vi "ACR_Connect_configTerminal.vi"() -> ()   [LabVIEW 2015]
uses:
  <vilib>/Instr/_visa.llb/VISA Configure Serial Port (Instr).vi
panel:
  in  "nPort":i32=28
  out "Speed Out":dbl
  out "Torque Out":dbl
  out "Running LED":bool
  in  "baud rate":u16(ring)=19200 items=["300"=300, "600"=600, "1200"=1200, "2400"=2400, "4800"=4800, "9600"=9600, "19200"=19200, "38400"=38400]
  in  "flow control":u16(ring) items=["None"=0, "XON/XOFF"=1, "RTS/CTS"=2, "DTR/DSR"=4]
  in  "stop bits":u16(ring)=10 items=["1.0"=10, "1.5"=15, "2.0"=20]
  in  "parity":u16(ring) items=["None", "Odd", "Even", "Mark", "Space"]
  in  "data bits":u16=8 min=5 max=8 step=1
  in  "VISA Refnum in":refnum<visa-resource-name>="COM5"
  in  "Reset Graph":bool
  in  "Sampling Time (s)":dbl=0.2
  out "Read result 2":dbl
  in  "Target":string="p12289"
  out "XY Graph":cluster{dbl[], dbl[]}[](graph)
  out "Read result":dbl
  out "Read error out":errorcluster
  in  "Read error in \n(no error)":errorcluster
  in  "Actual":string="p38144"
  in  "Move CMD":string="x/100"
  in  "OK Button":bool
  in  "Write String Array":string[](array[string])=["detach all", "new all", "clear", "attach master0", "attach slave0 axis0 \"x\"", "axis0 drive on"]
  out "Terminal Status":bool
  in  "ComACRServerLib.IChannel":refnum<k7>
  in  "bstrIP Property":string="192.168.10.40"
  out "Connect error out":errorcluster
  in  "Connect error in \n(no error)":errorcluster
  # "Ethernet Configuration"
  # "Command"
  # "Configure"
  # "detach all\nnew all\nclear\nattach master0\nattach slave0 axis0 \"x\"\naxis0 drive on"
  # "Read P Parameter"
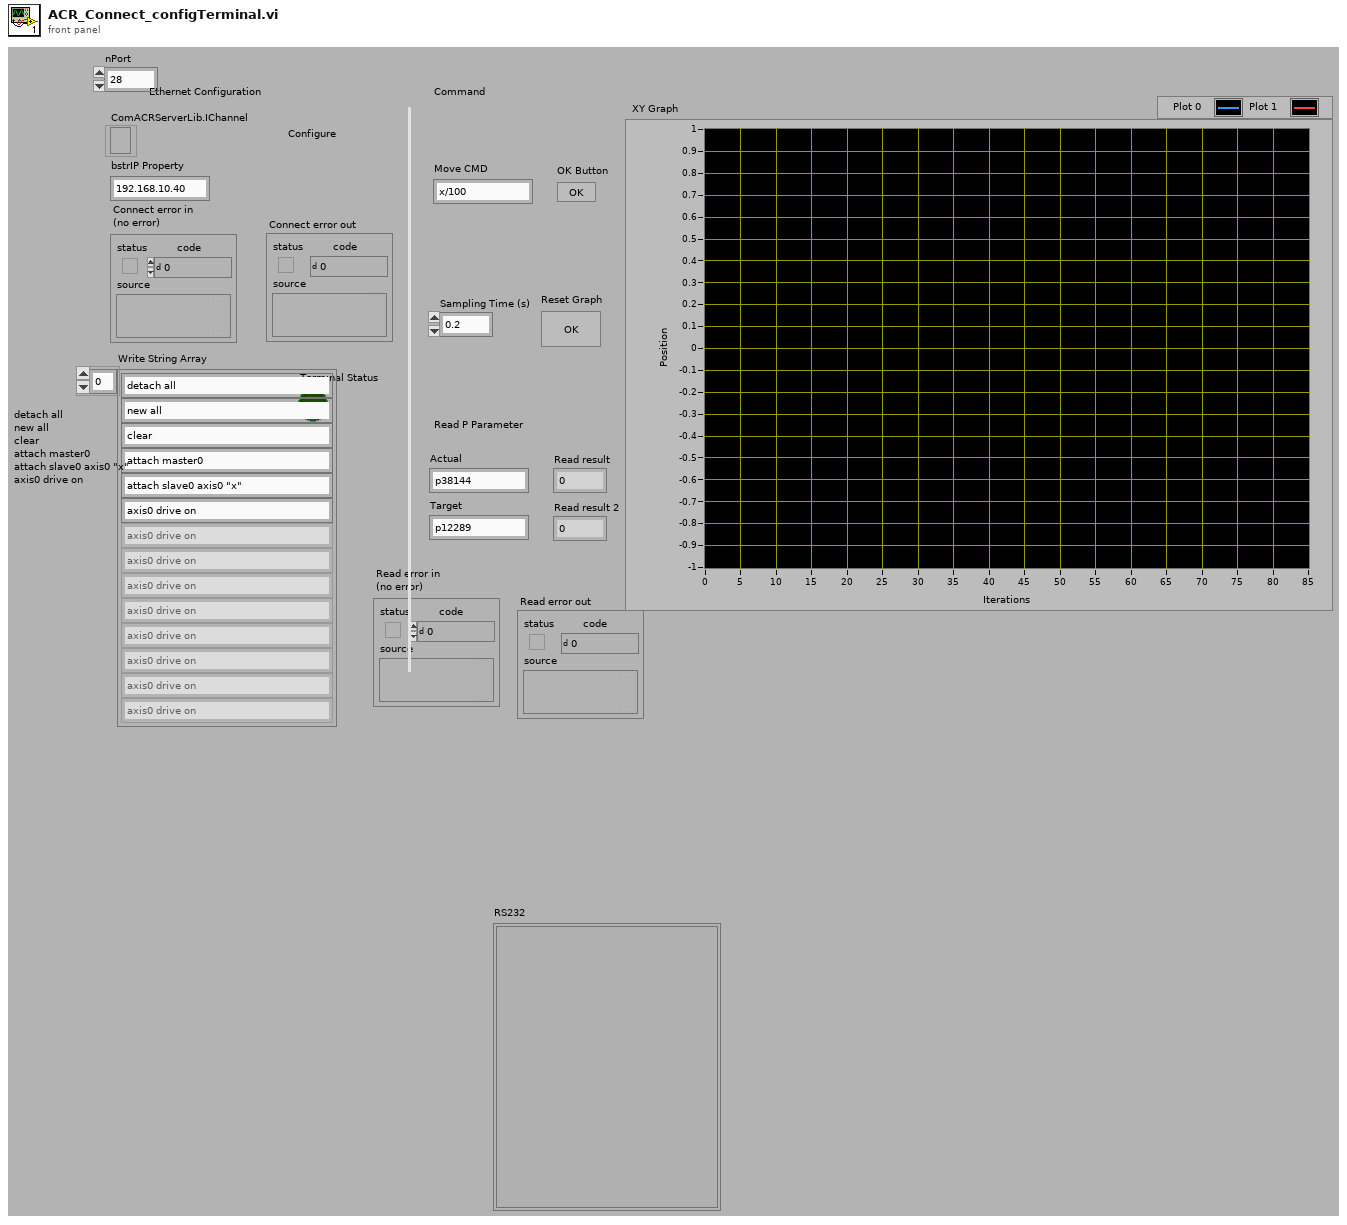
[diagram p1: front panel]
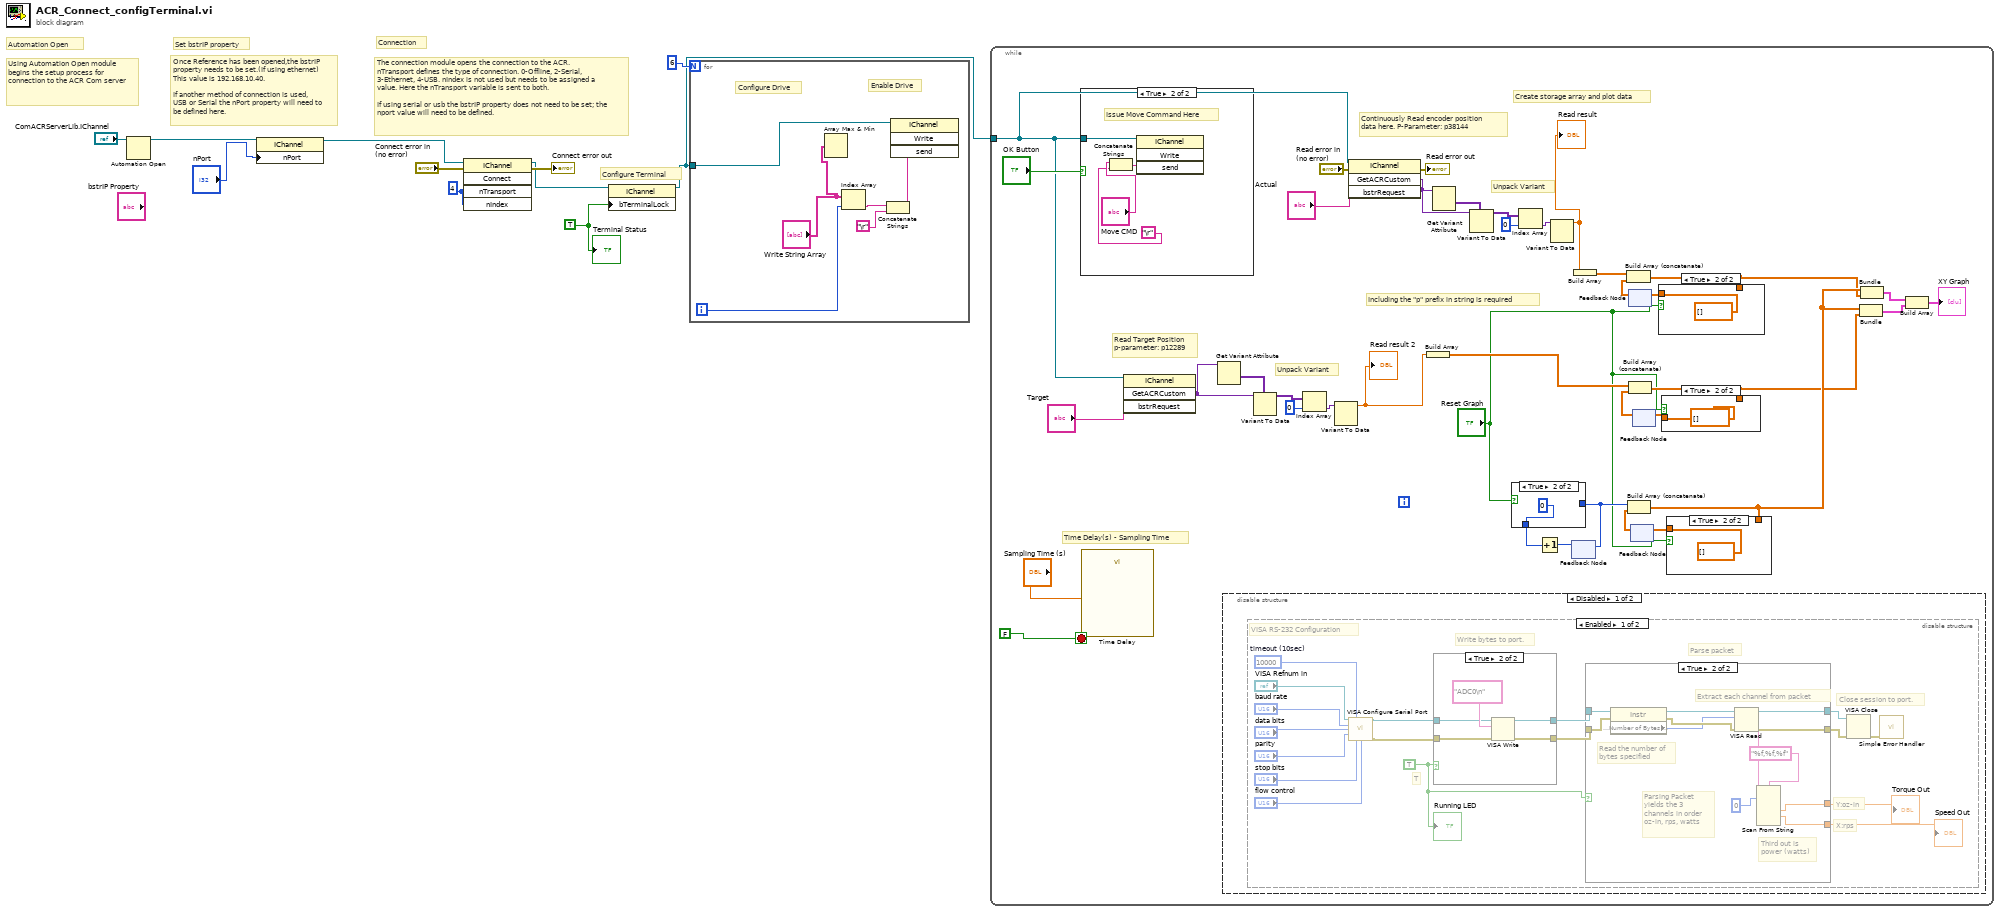
[diagram p0: block diagram]
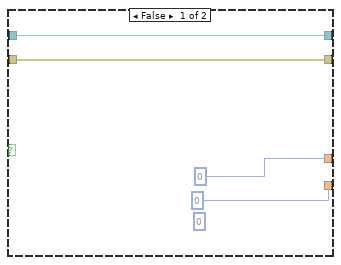
[diagram p2: hidden frame]
diagram:
  w3 = TRUE
  w8 = 4
  # "Configure Terminal"
  # "Using Automation Open module begins the setup process for connection to the ACR Com server"
  # "Automation Open"
  # "Once Reference has been opened,the bstrIP property needs to be set.(If using ethernet) This value is 192.168.10.40. \n\nIf another method of connection is used, USB or Serial the nPort property will need to be defined here."
  # "Set bstrIP property"
  # "The connection module opens the connection to the ACR. nTransport defines the type of connection. 0-Offline, 2-Serial, 3-Ethernet, 4-USB. nIndex is not used but needs to be assigned a value. Here the nTransport variable is sent to both.\n\nIf using serial or usb the bstrIP property does not need to be set; the nport value will need to be defined."
  # "Connection"
  n1 = Automation Open(Automation Refnum="ComACRServerLib.IChannel") -> (Automation Refnum=w7:refnum<k7>)  [unwired: 1 in, 3 out]
  n2 = property class="IChannel"(reference=w7, "nPort"="nPort") -> (reference out=w6:refnum<k7>)  [unwired: 1 in, 1 out]
  n3 = invoke class="IChannel" method="Connect"(reference=w6, error in="Connect error in \n(no error)", "nTransport"=w8, "nIndex"=w8) -> (reference out=w4:refnum<k7>, error out=→"Connect error out":errorcluster)  [unwired: 1 in, 3 out]
  n4 = property class="IChannel"(reference=w4, "bTerminalLock"=w3) -> (reference out=w2:refnum<k7>)  [unwired: 1 in, 1 out]
  n5 = for {
    N: 6 -> [_]
    tunnel: w2 -> [w12]
    i -> [w13]
    # "Enable Drive"
    # "Configure Drive"
    n6 = Array Max & Min(array="Write String Array") -> ()  [unwired: 4 out]
    n7 = Index Array(array="Write String Array", index=w13) -> (element=w16:string)
    n8 = Concatenate Strings(w16, "\r") -> (w17:string)
    n9 = invoke class="IChannel" method="Write"(reference=w12, "send"=w17) -> ()  [unwired: 2 in, 4 out]
  }
  n10 = while {
    tunnel: w2 -> [w41]
    stop <- FALSE stop-if-true
    # "Read Target Position\np-parameter: p12289"
    # "Unpack Variant"
    # "Time Delay(s) - Sampling Time"
    # "Create storage array and plot data"
    # "Continuously Read encoder position\ndata here. P-Parameter: p38144"
    # "Including the \"p\" prefix in string is required"
    # "Unpack Variant"
    n11 = case shown="True" "OK Button" {
      tunnel: w41 -> [_ w104]
      frame False {
      }
      frame True {
        # "Issue Move Command Here"
        n12 = Concatenate Strings("Move CMD", "\r") -> (w107:string)
        n13 = invoke class="IChannel" method="Write"(reference=w104, "send"=w107) -> ()  [unwired: 2 in, 4 out]
      }
    }
    n14 = call "Time Delay"("Delay Time (s)"="Sampling Time (s)") -> ()  [unwired: 1 in, 10 out]
    n15 = invoke class="IChannel" method="GetACRCustom"(reference=w41, "bstrRequest"="Target") -> ("GetACRCustom"=w39:variant)  [unwired: 2 in, 3 out]
    n16 = Get Variant Attribute(Variant=w39) -> (values=w40:variant[])  [unwired: 1 in, 5 out]
    n17 = disable-structure shown="Disabled" {
      frame Disabled {
        n18 = disable-structure shown="Enabled" {
          frame Enabled {
            w57 = TRUE
            w69 = u32 10000  # timeout (10sec)
            # "Parse packet"
            # "X:rps"
            # "Y:oz-in"
            # "Close session to port."
            # "T"
            # "Write bytes to port."
            # "VISA RS-232 Configuration"
            n19 = call-poly "VISA Configure Serial Port"("VISA resource name"="VISA Refnum in", "timeout (10sec)"=w69, "baud rate (9600)"="baud rate", "data bits (8)"="data bits", "parity (0:none)"="parity", "stop bits (10: 1 bit)"="stop bits", "flow control (0:none)"="flow control") -> ("VISA resource name out"=w66:refnum<visa-resource-name>, "error out"=w65:errorcluster)  [unwired: 1 in, 6 out]
            n20 = case shown="True" w57 {
              tunnel: [w90 w95] -> w58
              tunnel: w66 -> [w89 w93]
              tunnel: w65 -> [w90 w92]
              tunnel: [w89 w91] -> w59
              frame False {
              }
              frame True {
                n21 = VISA Write(VISA resource name=w93, write buffer="ADC0\n" ("string to write"), error in (no error)=w92) -> (VISA resource name out=w91:refnum<visa-resource-name>, error out=w95:errorcluster)  [unwired: 1 out]
              }
            }
            n22 = case shown="True" w57 {
              tunnel: w58 -> [w76 w84]
              tunnel: [w76 w88] -> w60
              tunnel: [w75 w87] -> w61
              tunnel: w59 -> [w75 w86]
              tunnel: [0 w79] -> w64
              tunnel: [0 w78] -> w63
              frame False {
                (unwired) 0
              }
              frame True {
                # "Parsing Packet\nyields the 3 \nchannels in order\noz-in, rps, watts"
                # "Third out is \npower (watts)"
                # "Extract each channel from packet"
                # "Read the number of bytes specified"
                n23 = property class="Instr"(reference=w86, error in=w84) -> (reference out=w85:refnum<visa-resource-name>, error out=w83:errorcluster, "Serial Settings:Number of Bytes at Serial Port"=w82:u32)
                n24 = VISA Read(VISA resource name=w85, byte count=w82, error in (no error)=w83) -> (VISA resource name out=w87:refnum<visa-resource-name>, read buffer=w77:string, error out=w88:errorcluster)  [unwired: 1 out]
                n25 = Scan From String(format string="%f,%f,%f", input string=w77, initial scan location=u32 0) -> (output 1=w79:dbl, output 2=w78:dbl)  [unwired: 1 in, 7 out]
              }
            }
            "Torque Out" <- w64
            "Speed Out" <- w63
            n26 = VISA Close(VISA resource name=w61, error in (no error)=w60) -> (error out=w62:errorcluster)
            n27 = call <vilib>:"Simple Error Handler.vi"("error in (no error)"=w62) -> ()  [unwired: 1 in, 8 out]
            "Running LED" <- w57
          }
          frame Disabled {
          }
        }
      }
      frame Enabled {
      }
    }
    n28 = Variant To Data(type=w40, Variant=w39) -> (data=w42:variant[])  [unwired: 1 in, 1 out]
    n29 = Index Array(array=w42, index=0) -> (element=w44:variant)
    n30 = Variant To Data(Variant=w44) -> (data=w35:dbl)  [unwired: 2 in, 1 out]
    "Read result 2" <- w35
    n31 = invoke class="IChannel" method="GetACRCustom"(reference=w41, error in="Read error in \n(no error)", "bstrRequest"="Actual") -> (error out=→"Read error out":errorcluster, "GetACRCustom"=w49:variant)  [unwired: 1 in, 2 out]
    n32 = Build Array(w35) -> (w33:dbl[])
    n33 = Get Variant Attribute(Variant=w49) -> (values=w50:variant[])  [unwired: 1 in, 5 out]
    n34 = Variant To Data(type=w50, Variant=w49) -> (data=w48:variant[])  [unwired: 1 in, 1 out]
    n35 = Index Array(array=w48, index=0) -> (element=w46:variant)
    n36 = Variant To Data(Variant=w46) -> (data=w36:dbl)  [unwired: 2 in, 1 out]
    "Read result" <- w36
    n37 = feedback #1() -> (w20:i32)  [unwired: 1 out]
    n38 = case shown="True" "Reset Graph" {
      tunnel: w20 -> [w96 _]
      tunnel: [w96 0] -> w19
      frame False {
      }
      frame True {
      }
    }
    n39 = Increment(x=w19) -> (x+1=w27:i32)
    n40 = feedback-in #1(w27) -> ()
    n41 = Build Array(w36) -> (w34:dbl[])
    n42 = feedback #2() -> (w31:dbl[])  [unwired: 1 out]
    n43 = Build Array (concatenate)(w34, w31) -> (w21:dbl[])
    n44 = feedback #3() -> (w29:dbl[])  [unwired: 1 out]
    n45 = Build Array (concatenate)(w20, w29) -> (w25:dbl[])
    n46 = feedback #4() -> (w30:dbl[])  [unwired: 1 out]
    n47 = Build Array (concatenate)(w33, w30) -> (w23:dbl[])
    n48 = case shown="True" "Reset Graph" {
      tunnel: [w98 dbl[] [] ("Array")] -> w22
      tunnel: w21 -> [w98 _]
      frame False {
      }
      frame True {
      }
    }
    n49 = feedback-in #2(w22) -> ()
    n50 = case shown="True" "Reset Graph" {
      tunnel: w23 -> [w100 _]
      tunnel: [w100 dbl[] [] ("Array")] -> w24
      frame False {
      }
      frame True {
      }
    }
    n51 = feedback-in #4(w24) -> ()
    n52 = case shown="True" "Reset Graph" {
      tunnel: [w102 dbl[] [] ("Array")] -> w26
      tunnel: w25 -> [w102 _]
      frame False {
      }
      frame True {
      }
    }
    n53 = feedback-in #3(w26) -> ()
    n54 = Bundle(w25, w23) -> (w28:cluster{dbl[], dbl[]})  [unwired: 1 out]
    n55 = Bundle(w25, w21) -> (w37:cluster{dbl[], dbl[]})  [unwired: 1 out]
    n56 = Build Array(w37, w28) -> (→"XY Graph":cluster{dbl[], dbl[]}[])
  }
  "Terminal Status" <- w3
